vi "Custom Test Static Ref.vi"(3 "Error In":errorcluster, 4 "Solution VI":path, 5 "User VI":path) -> (0 "Error Out":errorcluster, 2 "Results":T1={"Id"="", "Score"={"Status"=enum."Passed", "cpu_time"=-1, "max_memory"=-1, "style_score"=-1, "score0"="", "score1"="", "score2"="", "score3"="", "score4"="", "score5"=""}})   [LabVIEW 2013, in "VIChallenge.lvlib"]
doc: "This VI is a template for a custom users test. The User VI control will provide the absolute path to the VI to test. The solution VI control will provide the absolute path to the solution VI. The Results indicator should be populated with the results from testing the user submitted VI."
uses:
  <vilib>/LabVIEW Hacker/VIChallenge/Private/Grader/Type Defs/Grader Result.ctl
  <vilib>/LabVIEW Hacker/VIChallenge/Private/Type Defs/Database/Score.ctl
  <vilib>/LabVIEW Hacker/VIChallenge/Private/Grader/Type Defs/UTF Status.ctl
  <vilib>/LabVIEW Hacker/VIChallenge/VIChallenge.lvlib
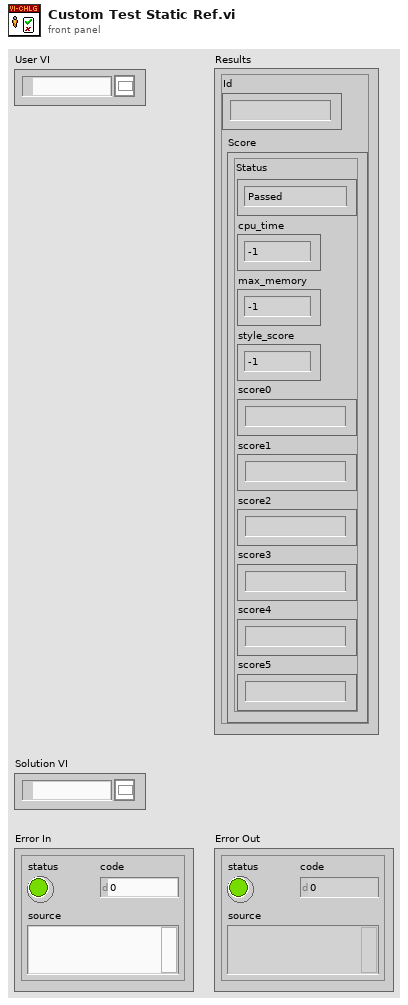
[diagram p1: front panel]
types:
  T1 = typedef "VIChallenge.lvlib/Grader Result.ctl" = cluster{"Id":string, "Score":T2}
  T2 = typedef "VIChallenge.lvlib/Score.ctl" = cluster{"Status":T3, "cpu_time":i32, "max_memory":i32, "style_score":i32, "score0":string, "score1":string, "score2":string, "score3":string, "score4":string, "score5":string}
  T3 = typedef "VIChallenge.lvlib/UTF Status.ctl" = enum16{"Null", "Passed", "Failed", "Error", "Skipped", "Not Processed"}
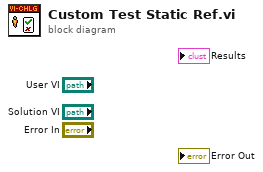
[diagram p0: block diagram]
diagram:
